vi "ModeSelect.vi"(10 "Buttons 2":bool[](array[boolean]), 11 "Buttons":bool[](array[boolean])) -> (3 "Numeric":i32)   [LabVIEW 2014]
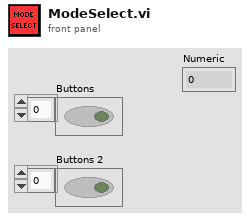
[diagram p1: front panel]
types:
  T1 = cluster{"Buttons[0]":bool, "Buttons[1]":bool, "Buttons[2]":bool, "Buttons[3]":bool, "Buttons[4]":bool, "Buttons[5]":bool, "Buttons[6]":bool, "Buttons[7]":bool, "Buttons[8]":bool}
  T2 = cluster{"Buttons 2[0]":bool, "Buttons 2[1]":bool, "Buttons 2[2]":bool, "Buttons 2[3]":bool, "Buttons 2[4]":bool, "Buttons 2[5]":bool, "Buttons 2[6]":bool, "Buttons 2[7]":bool, "Buttons 2[8]":bool}
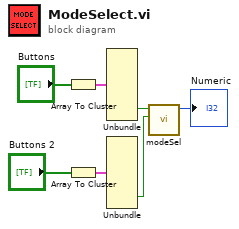
[diagram p0: block diagram]
diagram:
  n1 = Array To Cluster(array="Buttons") -> (cluster=w5:T1)
  n2 = Array To Cluster(array="Buttons 2") -> (cluster=w4:T2)
  n3 = Unbundle(w5) -> ("Buttons[7]"=w6:bool)  [unwired: 8 out]
  n4 = Unbundle(w4) -> ("Buttons 2[7]"=w7:bool)  [unwired: 8 out]
  n5 = call "modeSel.vi"("Buttons[7]"=w7, "Buttons[7] 2"=w6) -> ("Numeric"=→"Numeric":i32)  [unwired: 9 in]
